vi "test_alignBottomValidation.vi"(11 "Test Case In":refnum<class "AlignmentTests.lvclass">) -> (0 "error out":errorcluster, 3 "Test Case Out":refnum<class "AlignmentTests.lvclass">)   [LabVIEW 2023, in "AlignmentTests.lvclass"]
uses:
  AlignmentTests.lvclass
  <vilib>/Astemes/LUnit/Test Case.lvclass/Test Case.ctl
  <vilib>/Astemes/LUnit/Core/LUnit Test Case/Private/Append Fail Result.vi
  <vilib>/Astemes/LUnit/Core/LUnit Test Case/Private/Append Pass Result.vi
  <vilib>/Astemes/LUnit/Core/LUnit Test Case/Private/Run In UI.vi
  <vilib>/Utility/error.llb/Clear Errors.vi
  AlignmentTests.lvclass/AlignmentTests.ctl
  <vilib>/Astemes/LUnit/Test Case.lvclass
panel:
  in  "Numeric 3":dbl
  in  "Numeric 2":dbl
  in  "Numeric":dbl
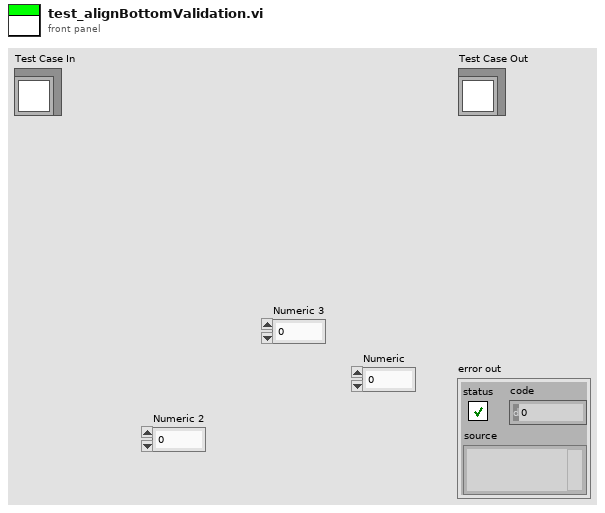
[diagram p1: front panel]
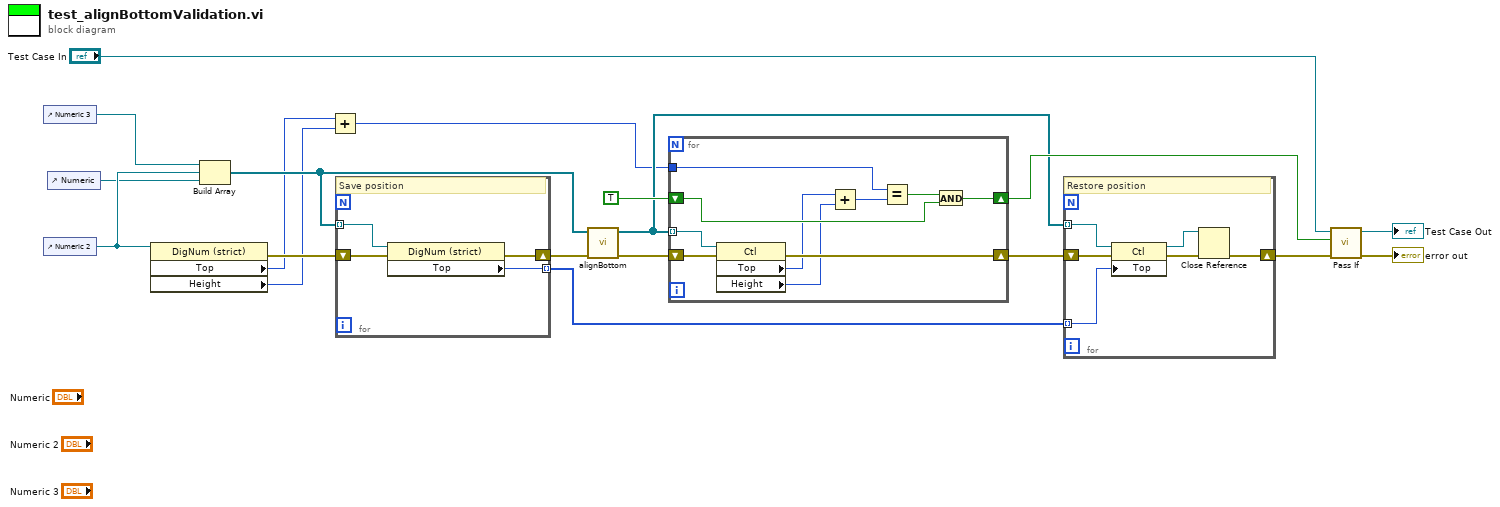
[diagram p0: block diagram]
diagram:
  n1 = control-ref of="Numeric 3"() -> (w16:refnum<vi>)
  n2 = control-ref of="Numeric 2"() -> (w15:refnum<vi>)
  n3 = control-ref of="Numeric"() -> (w14:refnum<vi>)
  n4 = property class="DigNum (strict)"(reference=w15) -> (error out=w10:errorcluster, "Top"=w2:i32, "Height"=w3:u32)  [unwired: 1 in, 1 out]
  n5 = Build Array(w16, w15, w14) -> (w5:refnum<vi>[])
  n6 = Add(x=w2, y=w3) -> (x+y=w1:u32)
  n7 = for {
    tunnel: w5 -> [w23] mode=indexing
    shift-right: [w21] -> w9
    shift-left: w10 -> [w22]
    tunnel: [w20] -> w6 mode=indexing
    # "Save position"
    n8 = property class="DigNum (strict)"(reference=w23, error in=w22) -> (error out=w21:errorcluster, "Top"=w20:i32)  [unwired: 1 out]
  }
  n9 = call "alignBottom.vi"("error in (no error)"=w9, "refs"=w5) -> ("error out"=w11:errorcluster, "refs(dup)"=w4:refnum<vi>[])  [unwired: 8 in]
  n10 = for {
    tunnel: w4 -> [w33] mode=indexing
    tunnel: w1 -> [w32]
    shift-right: [w30] -> w12
    shift-left: TRUE -> [w29]
    shift-right: [w27] -> w7
    shift-left: w11 -> [w28]
    n11 = property class="Ctl"(reference=w33, error in=w28) -> (error out=w27:errorcluster, "Top"=w25:i32, "Height"=w26:u32)  [unwired: 1 out]
    n12 = Add(x=w25, y=w26) -> (x+y=w24:u32)
    n13 = Equal?(x=w32, y=w24) -> (x = y?=w31:bool)
    n14 = And(x=w31, y=w29) -> (x .and. y?=w30:bool)
  }
  n15 = for {
    tunnel: w4 -> [w39] mode=indexing
    shift-right: [w35] -> w8
    shift-left: w7 -> [w38]
    tunnel: w6 -> [w36] mode=indexing
    # "Restore position"
    n16 = property class="Ctl"(reference=w39, error in=w38, "Top"=w36) -> (reference out=w34:refnum<vi>, error out=w37:errorcluster)
    n17 = Close Reference(reference=w34, error in (no error)=w37) -> (error out=w35:errorcluster)
  }
  n18 = call <vilib>:"Pass If.vi"("error in (no error)"=w8, "Pass?"=w12, "LUnit Test Case In"="Test Case In") -> ("error out"=→"error out":errorcluster, "LUnit Test Case Out"=→"Test Case Out":refnum<class "AlignmentTests.lvclass">)  [unwired: 7 in]
